vi "test-tirf-lock.vi"() -> ()   [LabVIEW 2014]
panel:
  out "Calibration curve":cluster{ext[], dbl[]}(graph)
  out "Error Out":errorcluster
  in  "?":bool
  out "Power Intensity":dbl(graph)
  out "Intensity 2":cluster{"X position":dbl, "Y position":dbl}(graph)
  in  "stop":bool
  in  "Go?":bool
  out "Supply Voltage":dbl format="%#_13g"
  in  "number of readings\n to average":i32=1
  in  "Mode":enum16{"Start", "Read", "End"}(ring)=enum."Read"
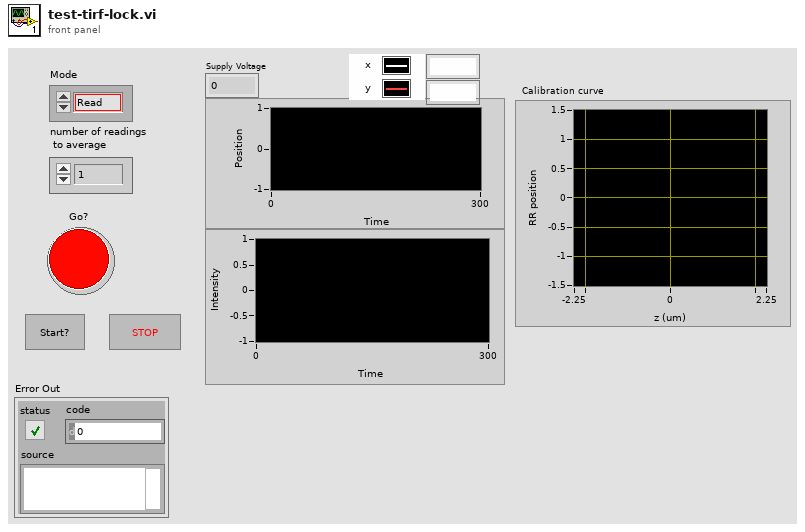
[diagram p1: front panel]
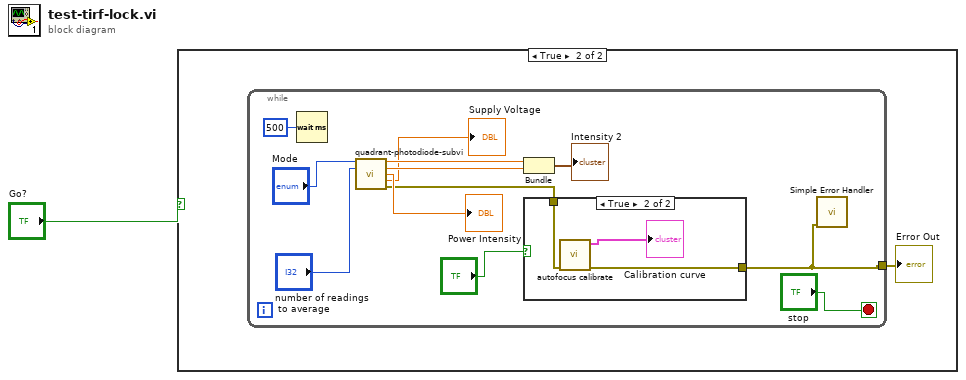
[diagram p0: block diagram]
diagram:
  n1 = case shown="True" "Go?" {
    frame False {
    }
    frame True {
      n2 = while {
        tunnel: [w3] -> w2
        stop <- "stop" stop-if-true
        n3 = Wait (ms)(milliseconds to wait=u32 500) -> ()  [unwired: 1 out]
        n4 = call "quadrant-photodiode-subvi.vi"("Mode"="Mode", "number of readings\n to average"="number of readings\n to average") -> ("X-position"=w9:dbl, "Y-position"=w10:dbl, "Power"=→"Power Intensity":dbl, "Supply Voltage"=→"Supply Voltage":dbl, "Error Out"=w4:errorcluster)  [unwired: 9 in]
        n5 = Bundle("X-position"=w9, "Y-position"=w10) -> (→"Intensity 2":cluster{"X-position":dbl, "Y-position":dbl})  [unwired: 1 in]
        n6 = case shown="True" "?" {
          tunnel: w4 -> [w15 w18]
          tunnel: [w15 w17] -> w3
          frame False {
          }
          frame True {
            n7 = call "autofocus calibrate.vi"("Error In"=w18) -> ("Error Out"=w17:errorcluster, "Cal. curve"=→"Calibration curve":cluster{ext[], dbl[]})  [unwired: 8 in, 1 out]
          }
        }
        n8 = call <vilib>:"Simple Error Handler.vi"("error in (no error)"=w3) -> ()  [unwired: 4 in, 5 out]
      }
      "Error Out" <- w2
    }
  }
